vi "DownsampleStage2_5772.vi"(8 "valid in":bool, 9 "reset":bool, 11 "Data in":fxp<+/-,16,14>[](array[numeric])=[0.0, 0.0, 0.0, 0.0]) -> (0 "valid out":bool, 3 "data out":fxp<+/-,16,14>[](array[numeric]))   [LabVIEW 2013]
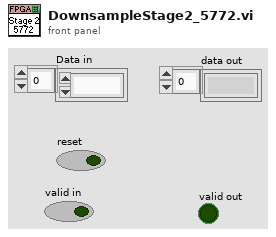
[diagram p1: front panel]
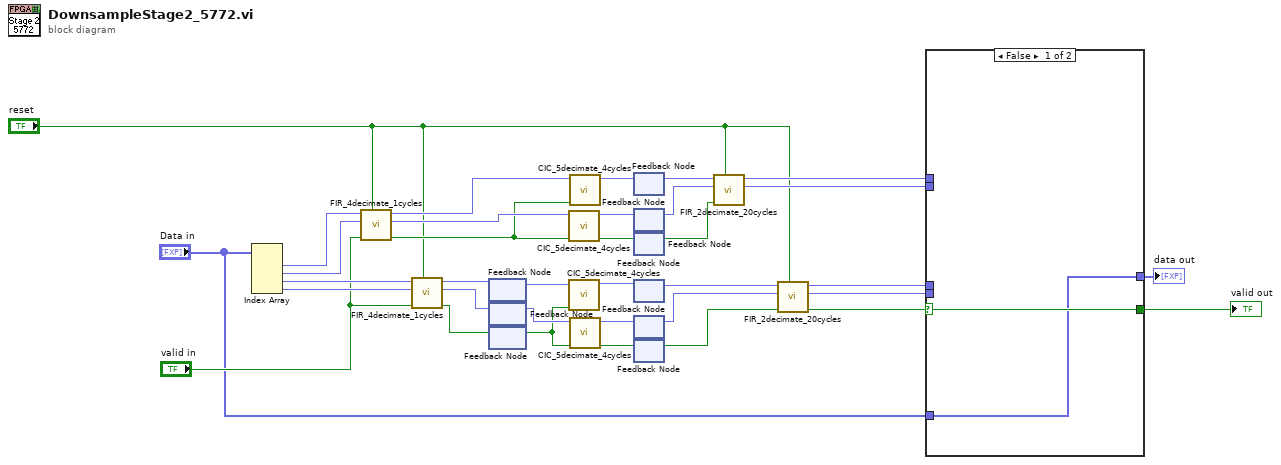
[diagram p0: block diagram]
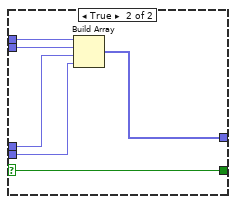
[diagram p2: hidden frame]
diagram:
  n1 = Index Array(array="Data in") -> (element #1=w33:fxp<+/-,16,14>, element #2=w32:fxp<+/-,16,14>, element #3=w31:fxp<+/-,16,14>, element #4=w30:fxp<+/-,16,14>)  [unwired: 4 in]
  n2 = call "FIR_4decimate_1cycles.vi"("reset"="reset", "valid in"="valid in", "Q in"=w32, "I in"=w33) -> ("valid out"=w20:bool, "Q out"=w21:fxp<+/-,16,14>, "I out"=w22:fxp<+/-,16,14>)  [unwired: 4 in, 1 out]
  n3 = call "FIR_4decimate_1cycles.vi"("reset"="reset", "valid in"="valid in", "Q in"=w30, "I in"=w31) -> ("valid out"=w26:bool, "Q out"=w27:fxp<+/-,16,14>, "I out"=w28:fxp<+/-,16,14>)  [unwired: 4 in, 1 out]
  n4 = feedback #1() -> (w25:fxp<+/-,16,14>)  [unwired: 1 in]
  n5 = feedback-in #1(w28) -> ()
  n6 = feedback #2() -> (w24:fxp<+/-,16,14>)  [unwired: 1 in]
  n7 = feedback-in #2(w27) -> ()
  n8 = feedback #3() -> (w23:bool)  [unwired: 1 in]
  n9 = feedback-in #3(w26) -> ()
  n10 = call "CIC_5decimate_4cycles.vi"("valid in"=w20, "Data in"=w21) -> ("valid out"=w15:bool, "Data out"=w17:fxp<+/-,16,14>)  [unwired: 7 in, 1 out]
  n11 = call "CIC_5decimate_4cycles.vi"("valid in"=w23, "Data in"=w25) -> ("Data out"=w10:fxp<+/-,16,14>)  [unwired: 7 in, 2 out]
  n12 = call "CIC_5decimate_4cycles.vi"("valid in"=w20, "Data in"=w22) -> ("Data out"=w19:fxp<+/-,16,14>)  [unwired: 7 in, 2 out]
  n13 = call "CIC_5decimate_4cycles.vi"("valid in"=w23, "Data in"=w24) -> ("valid out"=w8:bool, "Data out"=w9:fxp<+/-,16,14>)  [unwired: 7 in, 1 out]
  n14 = feedback #4() -> (w18:fxp<+/-,16,14>)  [unwired: 1 in]
  n15 = feedback-in #4(w19) -> ()
  n16 = feedback #5() -> (w16:fxp<+/-,16,14>)  [unwired: 1 in]
  n17 = feedback-in #5(w17) -> ()
  n18 = feedback #6() -> (w14:bool)  [unwired: 1 in]
  n19 = feedback-in #6(w15) -> ()
  n20 = feedback #7() -> (w11:fxp<+/-,16,14>)  [unwired: 1 in]
  n21 = feedback-in #7(w10) -> ()
  n22 = feedback #8() -> (w12:fxp<+/-,16,14>)  [unwired: 1 in]
  n23 = feedback-in #8(w9) -> ()
  n24 = feedback #9() -> (w13:bool)  [unwired: 1 in]
  n25 = feedback-in #9(w8) -> ()
  n26 = call "FIR_2decimate_20cycles.vi"("reset"="reset", "valid in"=w14, "Q in"=w16, "I in"=w18) -> ("Q out"=w6:fxp<+/-,16,14>, "I out"=w7:fxp<+/-,16,14>)  [unwired: 4 in, 2 out]
  n27 = call "FIR_2decimate_20cycles.vi"("reset"="reset", "valid in"=w13, "Q in"=w12, "I in"=w11) -> ("valid out"=w3:bool, "Q out"=w4:fxp<+/-,16,14>, "I out"=w5:fxp<+/-,16,14>)  [unwired: 4 in, 1 out]
  n28 = case shown="False" w3 {
    selector: w3 -> [w37 w43]
    tunnel: w7 -> [_ w42]
    tunnel: w6 -> [_ w41]
    tunnel: w5 -> [_ w39]
    tunnel: w4 -> [_ w40]
    tunnel: [w36 w38] -> w35
    tunnel: [w37 w43] -> w34
    tunnel: "Data in" -> [w36 _]
    frame False {
    }
    frame True {
      n29 = Build Array(w42, w41, w39, w40) -> (w38:fxp<+/-,16,14>[])
    }
  }
  "data out" <- w35
  "valid out" <- w34
